vi "Read TCP.vi"(8 "error in (no error)":errorcluster, 9 "Timeout (ms)":i32, 10 "Bytes to Read":i32=1, 11 "Telnet V2 in":refnum<class "UDP.lvclass">) -> (0 "error out":errorcluster, 2 "Data Out":string, 3 "Telnet V2 out":refnum<class "UDP.lvclass">)   [LabVIEW 2018]
uses:
  UDP.lvclass
  C:/AME Test Engineering/LabVIEW/PPLs/LiDAR/Parent/LiDAR.lvlibp/LiDAR.lvclass
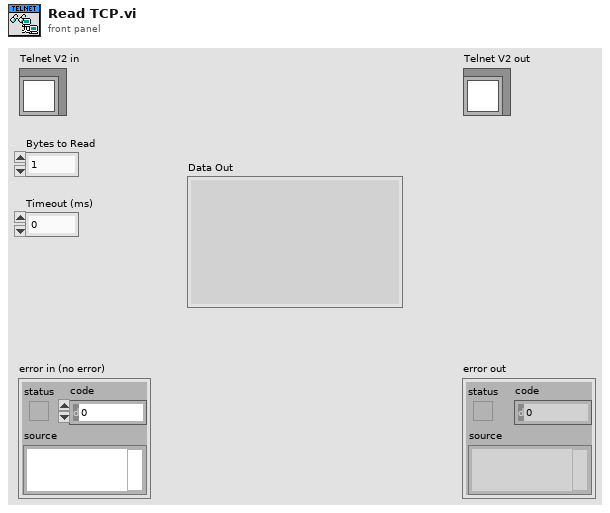
[diagram p1: front panel]
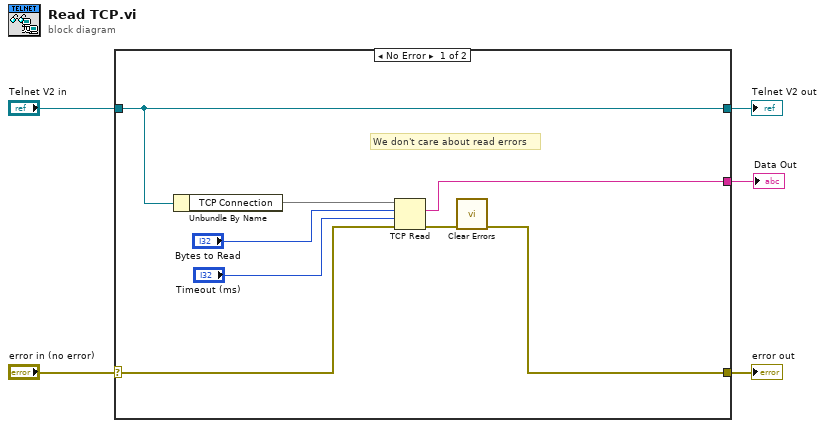
[diagram p0: block diagram]
diagram:
  n1 = case shown="No Error" "error in (no error)" {
    selector: "error in (no error)" -> [w9 w15]
    tunnel: [w7 w15] -> w4
    tunnel: [w13 w14] -> w2
    tunnel: "Telnet V2 in" -> [w13 w14]
    tunnel: [w6 _] -> w1
    frame No Error {
      # "We don't care about read errors"
      n2 = Unbundle By Name(w13) -> ("TCP Connection"=w12)
      n3 = TCP Read(connection ID=w12, bytes to read="Bytes to Read", error in (no error)=w9, 9:"Timeout (ms)") -> (data out=w6:string, error out=w8:errorcluster)  [unwired: 1 in, 1 out]
      n4 = call <vilib>:"Clear Errors.vi"("error in (no error)"=w8) -> ("error out"=w7:errorcluster)  [unwired: 5 in, 1 out]
    }
    frame Error {
    }
  }
  "error out" <- w4
  "Telnet V2 out" <- w2
  "Data Out" <- w1
